vi "đọc biển số xe 2.vi"() -> ()   [LabVIEW 2020]
uses:
  <vilib>/userdefined/High Color/IMAQdx.ctl
  <vilib>/vision/driver/NI_Vision_Acquisition_Software.lvlib
  <vilib>/vision/NI_Vision_Development_Module.lvlib
panel:
  in  "File Path":path
  in  "Rectangle":T1 {"Rotation" min=-90.0 max=90.0 step=1.0 format="%.2f"; "Left" scale=0.0..1024.0; "Right" scale=0.0..1024.0}
  out "Image":T2(plugin-control)
  out "Read String":string
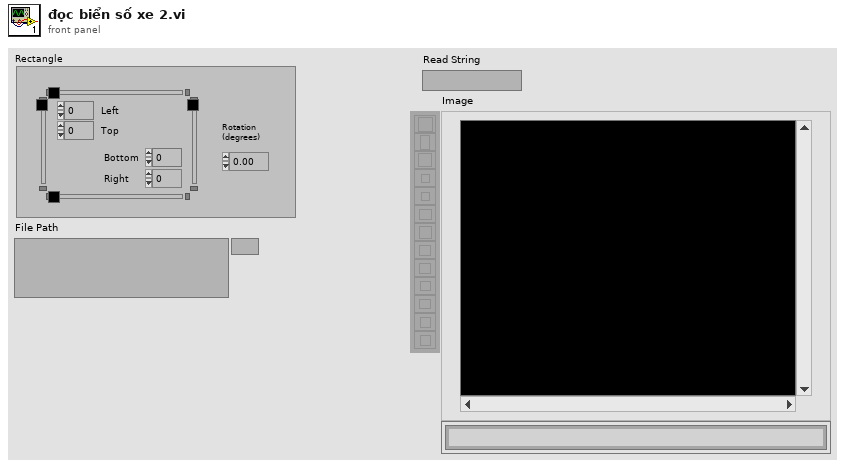
[diagram p1: front panel]
types:
  T1 = typedef "IMAQ Rectangle" = cluster{"Left":i32, "Top":i32, "Right":i32, "Bottom":i32, "Rotation":dbl}
  T2 = typedef "IMAQ Image.ctl" = refnum<image>
  T3 = typedef "IMAQdx.ctl" = refnum<k21>
  T4 = typedef "IMAQ OCR Session.ctl" = refnum<k1>
  T5 = typedef "ROI Descriptor" = cluster{"Global Rectangle":i32[], "Contours":cluster{"ID":enum32{"External", "Internal"}, "Type":u32, "Coordinates":i32[]}[]}
  T6 = cluster{"Global Rectangle":i32[], "Contours":cluster{"ID":enum32{"External", "Internal"}, "Type":u32, "Coordinates":i32[]}[]}
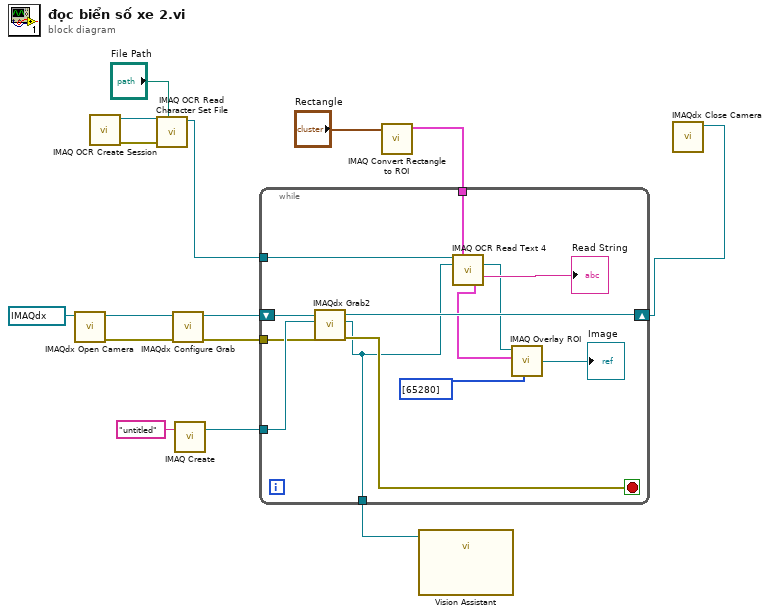
[diagram p0: block diagram]
diagram:
  n1 = call <vilib>:"IMAQdx Open Camera.vi"("Session In"=T3 "cam2") -> ("error out"=w14:errorcluster, "Session Out"=w15:T3)  [unwired: 9 in]
  n2 = call "IMAQ OCR Create Session"() -> ("error out"=w5:errorcluster, "IMAQ OCR Session"=w6:T4)  [unwired: 10 in]
  n3 = call "IMAQ OCR Read Character Set File"("File Path"="File Path", "error in (no error)"=w5, "IMAQ OCR Session"=w6) -> ("IMAQ OCR Session (dup)"=w4:T4)  [unwired: 6 in, 2 out]
  n4 = call <vilib>:"IMAQdx Configure Grab.vi"("error in"=w14, "Session In"=w15) -> ("error out"=w11:errorcluster, "Session Out"=w13:T3)  [unwired: 8 in]
  n5 = call "IMAQ Create"("Image Name"="untitled") -> ("New Image"=w12:T2)  [unwired: 4 in, 1 out]
  n6 = call "IMAQ Convert Rectangle to ROI"("Rectangle"="Rectangle") -> ("ROI Descriptor"=w3:T5)  [unwired: 8 in, 1 out]
  n7 = while {
    tunnel: w12 -> [w27]
    tunnel: w11 -> [w26]
    tunnel: [w16] -> w8
    tunnel: w4 -> [w21]
    tunnel: w3 -> [w20]
    shift-right: [w24] -> w7
    shift-left: w13 -> [w28]
    stop <- w17 stop-if-true
    n8 = call <vilib>:"IMAQdx Grab2.vi"("error in"=w26, "Image In"=w27, "Session In"=w28) -> ("error out"=w17:errorcluster, "Image Out"=w16:T2, "Session Out"=w24:T3)  [unwired: 5 in, 1 out]
    n9 = call "IMAQ OCR Read Text 4"("IMAQ OCR Session"=w21, "ROI Descriptor"=w20, "Image"=w16) -> ("Image (dup)"=w18:T2, "Read String"=→"Read String":string, "ROI Bounding Characters"=w22:T6)  [unwired: 6 in, 4 out]
    n10 = call "IMAQ Overlay ROI"("Colors (Green)"=u32[] [65280], "ROI Descriptor"=w22, "Image"=w18) -> ("Image Out"=→"Image":T2)  [unwired: 7 in, 1 out]
  }
  n11 = call "Vision Assistant"("Image In"=w8) -> ()  [unwired: 25 in, 2 out]
  n12 = call <vilib>:"IMAQdx Close Camera.vi"("Session In"=w7) -> ()  [unwired: 10 in, 1 out]
